vi "GetAxisButton.vi"(6 "coarseFactor":dbl=0.01, 7 "fastFactor":dbl=0.5, 8 "error in (no error)":errorcluster, 10 "timeout(s)":u32=30, 11 "Joystick in":refnum<class "Joystick.lvclass">) -> (0 "error out":errorcluster, 2 "AxisStep":dbl[](array[numeric]), 3 "Joystick out":refnum<class "Joystick.lvclass">, 4 "lock":bool, 5 "Coarse":bool)   [LabVIEW 2014, in "Joystick.lvclass"]
uses:
  Joystick.lvclass
  Joystick.lvclass/Joystick.ctl
  <vilib>/Utility/inputDevices.llb/joystickAcquire.vi
panel:
  in  "timeOffset":dbl
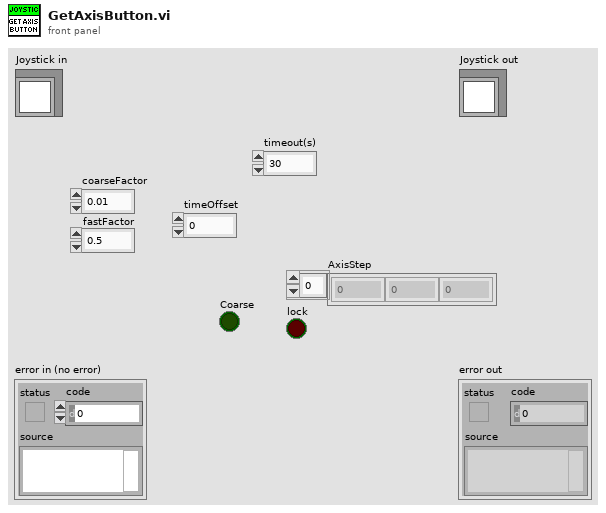
[diagram p1: front panel]
types:
  T1 = cluster{"X axis":i32, "Y axis":i32, "Z axis":i32, "X axis rotation":i32, "Y axis rotation":i32, "Z axis rotation":i32, "U axis":i32, "V axis":i32}
  T2 = cluster{"button 1":bool, "button 2":bool, "button 3":bool, "button 4":bool, "button 5":bool, "button 6":bool, "button 7":bool, "button 8":bool, "button 9":bool, "button 10":bool, "button 11":bool, "button 12":bool, "button 13":bool, "button 14":bool, "button 15":bool, "button 16":bool, "button 17":bool, "button 18":bool, "button 19":bool, "button 20":bool, "button 21":bool, "button 22":bool, "button 23":bool, "button 24":bool, "button 25":bool, "button 26":bool, "button 27":bool, "button 28":bool, "button 29":bool, "button 30":bool, "button 31":bool, "button 32":bool}
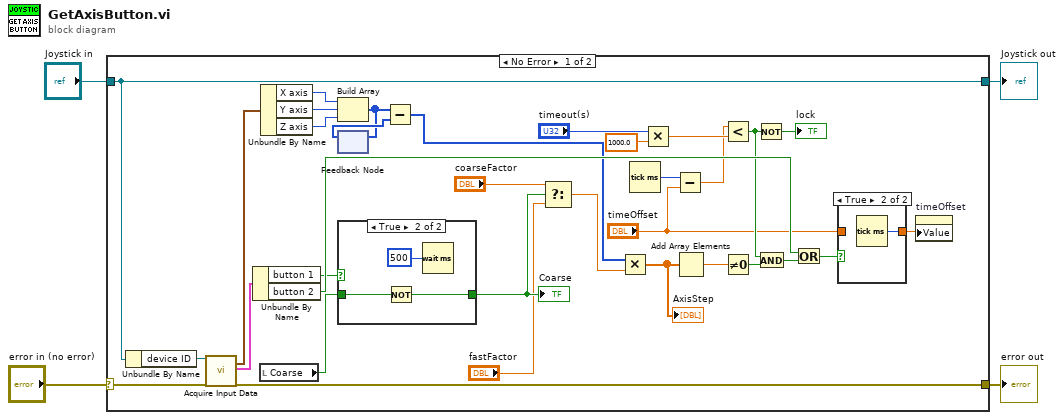
[diagram p0: block diagram]
diagram:
  n1 = case shown="No Error" "error in (no error)" {
    selector: "error in (no error)" -> [w35 w45]
    tunnel: [w34 w45] -> w3
    tunnel: [w37 w44] -> w1
    tunnel: "Joystick in" -> [w37 w44]
    frame No Error {
      n2 = Unbundle By Name(w37) -> ("device ID"=w36:refnum<k1>)
      n3 = call-poly <vilib>:"Acquire Input Data.vi"("device ID"=w36, "error in (no error)"=w35) -> ("axis info"=w9:T1, "button info"=w8:T2, "error out"=w34:errorcluster)  [unwired: 13 in, 2 out]
      n4 = Unbundle By Name(w8) -> ("button 1"=w31:bool, "button 2"=w33:bool)
      n5 = local read "Coarse"() -> (w5:bool)
      n6 = Unbundle By Name(w9) -> ("X axis"=w13:i32, "Y axis"=w12:i32, "Z axis"=w11:i32)
      n7 = Build Array(w13, w12, w11) -> (w10:i32[])
      n8 = feedback #1() -> (w14:i32[])  [unwired: 1 in]
      n9 = feedback-in #1(w10) -> ()
      n10 = case shown="True" w31 {
        tunnel: w5 -> [w38 w41]
        tunnel: [w38 w40] -> w32
        frame False {
        }
        frame True {
          n11 = Not(x=w41) -> (.not. x?=w40:bool)
          n12 = Wait (ms)(milliseconds to wait=u32 500) -> ()  [unwired: 1 out]
        }
      }
      "Coarse" <- w32
      n13 = Subtract(x=w10, y=w14) -> (x-y=w15:i32[])
      n14 = Select(t="coarseFactor", s=w32, f="fastFactor") -> (s? t:f=w25:dbl)
      n15 = Multiply(x=w15, y=w25) -> (x*y=w19:dbl[])
      "AxisStep" <- w19
      n16 = Tick Count (ms)() -> (millisecond timer value=w16:u32)
      n17 = Multiply(x="timeout(s)", y=1000.0) -> (x*y=w28:dbl)
      n18 = Subtract(x=w16, y="timeOffset") -> (x-y=w17:dbl)
      n19 = Add Array Elements(numeric array=w19) -> (sum=w18:dbl)
      n20 = Less?(x=w17, y=w28) -> (x < y?=w23:bool)
      n21 = Not Equal To 0?(x=w18) -> (x != 0?=w20:bool)
      n22 = Not(x=w23) -> (.not. x?=→"lock":bool)
      n23 = And(x=w23, y=w20) -> (x .and. y?=w21:bool)
      n24 = Or(x=w33, y=w21) -> (x .or. y?=w22:bool)
      n25 = case shown="True" w22 {
        tunnel: [w42 w43] -> w6
        tunnel: "timeOffset" -> [w42 _]
        frame False {
        }
        frame True {
          n26 = Tick Count (ms)() -> (millisecond timer value=w43:u32)
        }
      }
      n27 = property on="timeOffset" class="DigNum (strict)"("Value"=w6) -> ()  [unwired: 2 in, 2 out]
    }
    frame Error {
    }
  }
  "error out" <- w3
  "Joystick out" <- w1
